vi "startTestSeries.vi"(0 "State in":refnum<class "State.lvclass">, 1 "Model in":refnum<class "Model.lvclass">, 2 "Serial Number":string, 3 "Operator":string, 4 "Comments":string, 5 "error in (no error)":errorcluster) -> (14 "State out":refnum<class "State.lvclass">, 15 "Model out":refnum<class "Model.lvclass">, 19 "error out":errorcluster)   [LabVIEW 2015, in "State.lvclass"]
uses:
  State.lvclass
  Model/Model/Model.lvclass
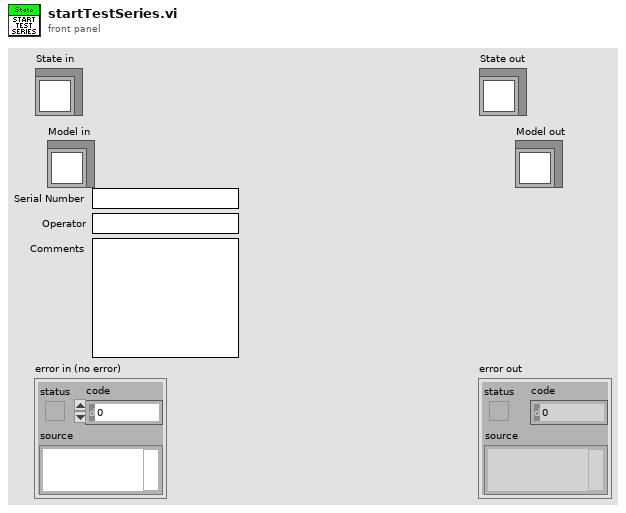
[diagram p1: front panel]
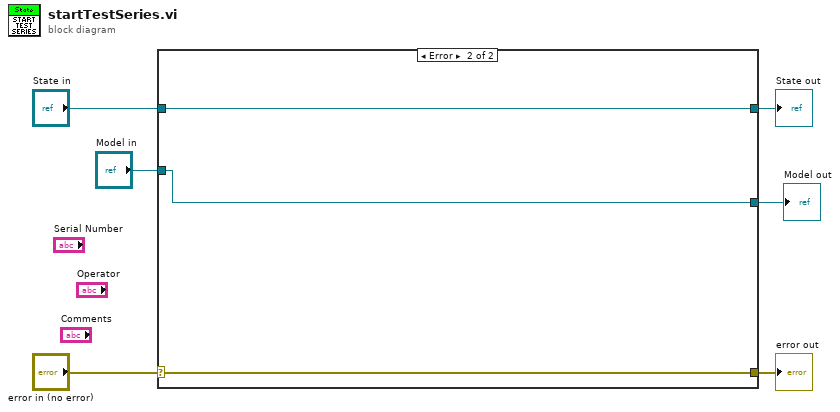
[diagram p0: block diagram]
diagram:
  n1 = case shown="Error" "error in (no error)" {
    selector: "error in (no error)" -> [w8 w12]
    tunnel: [w8 w12] -> w5
    tunnel: [w9 w11] -> w3
    tunnel: "State in" -> [w9 w11]
    tunnel: "Model in" -> [w7 w10]
    tunnel: [w7 w10] -> w1
    frame No Error {
      # "Wire the error cluster across even in the \"No Error\"\ncase so that warnings get propagated."
    }
    frame Error {
    }
  }
  "error out" <- w5
  "State out" <- w3
  "Model out" <- w1
